vi "CursorReturnForce.vi"(6 "Enable":bool, 8 "ReturnForce":dbl, 9 "Test Name":string(combo)="WDW", 10 "XYGRF_Up":refnum<vi>, 11 "XYGRF_Down":refnum<vi>) -> ()   [LabVIEW 2017]
panel:
  out "DoorLockGraph 2":cluster{"Y":dbl[], "Y":dbl[]}[](graph)
  out "DoorLockGraph":cluster{"Y":dbl[], "Y":dbl[]}[](graph)
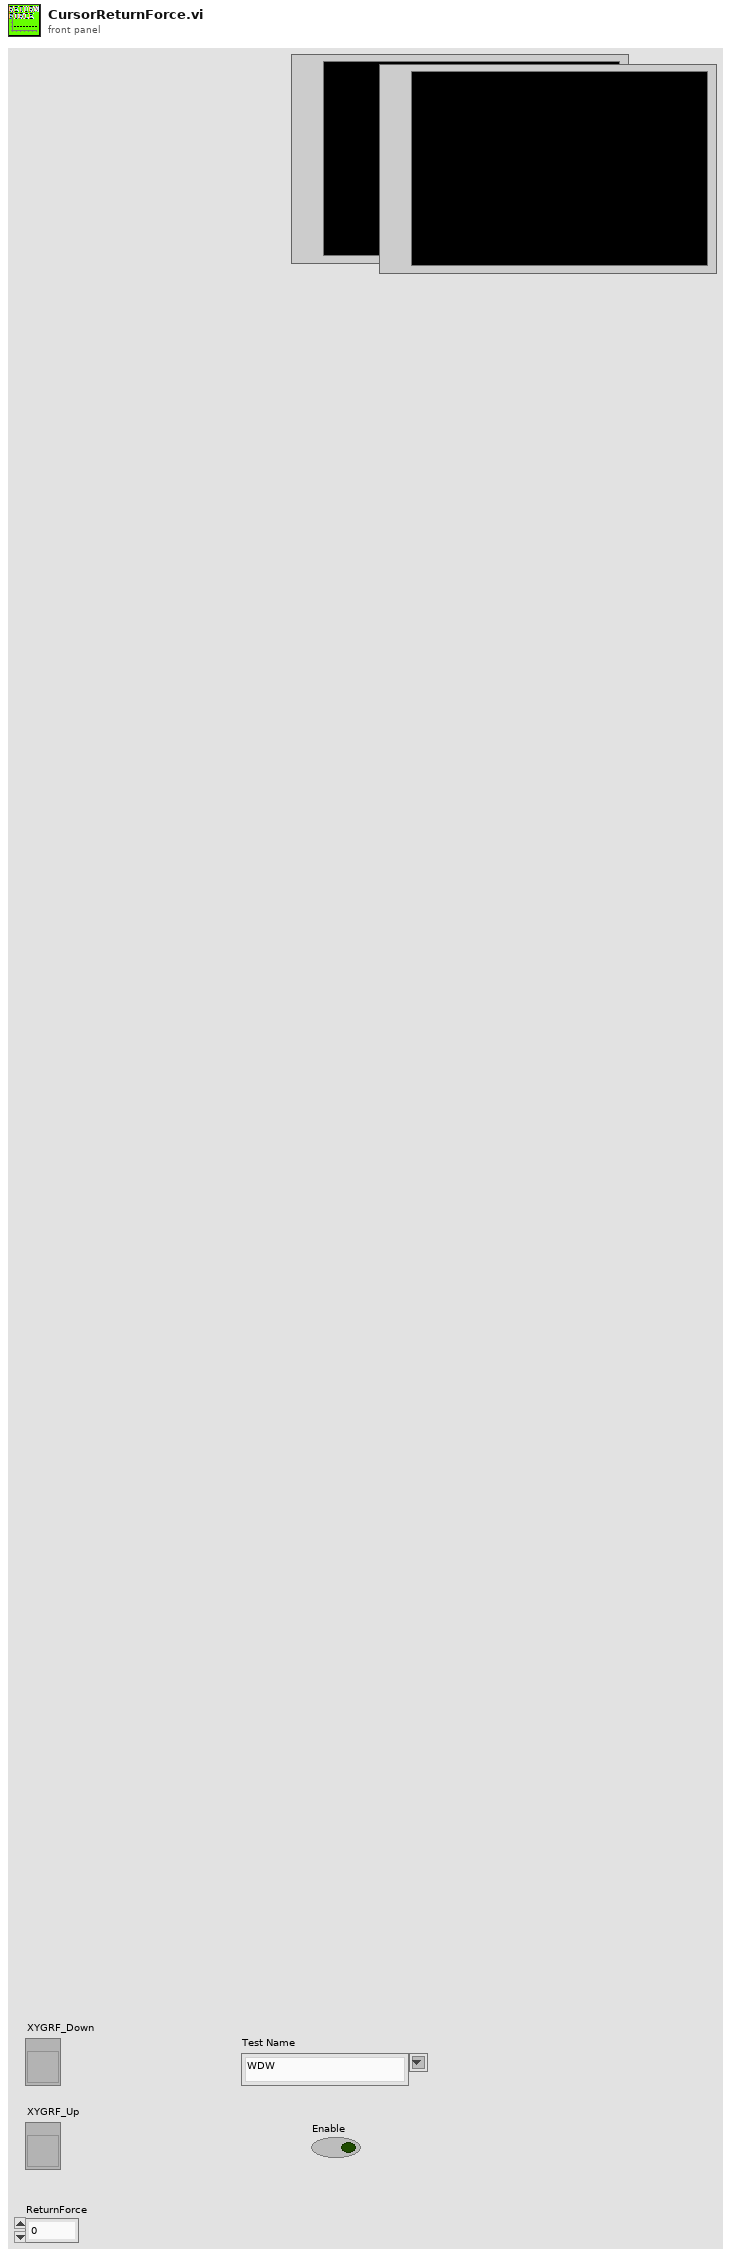
[diagram p1: front panel]
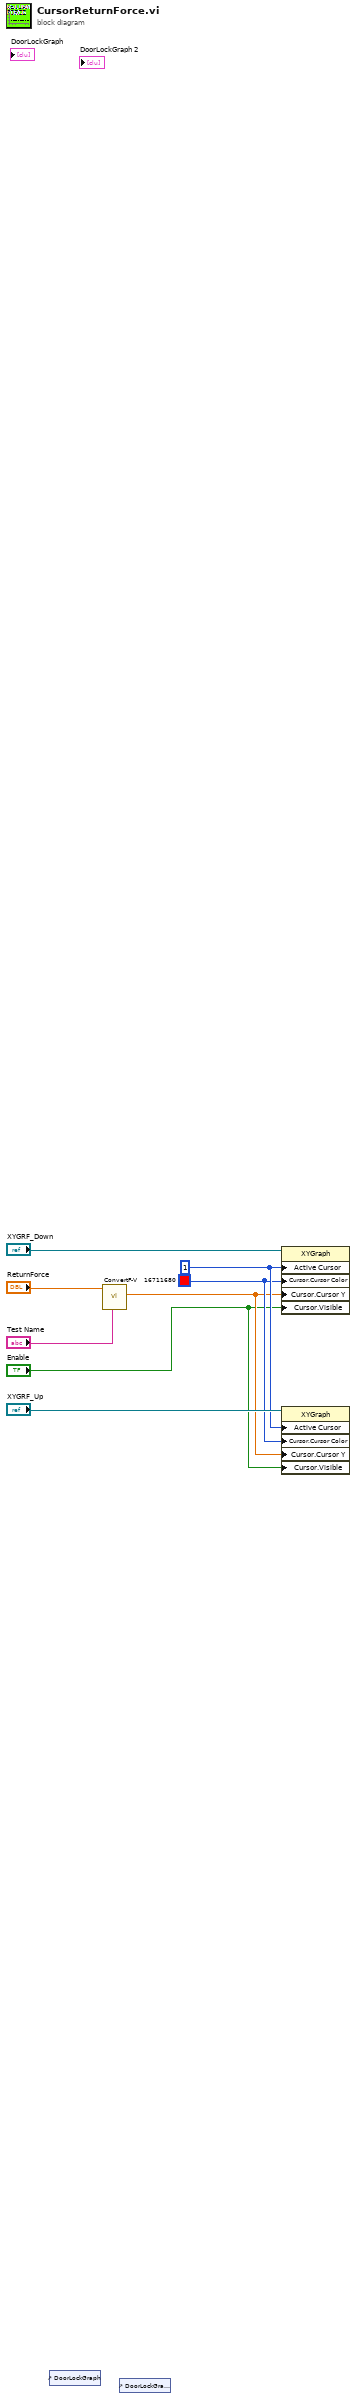
[diagram p0: block diagram]
diagram:
  w3 = u32 16711680
  w4 = u32 1 ("Active Cursor")
  n1 = control-ref of="DoorLockGraph"() -> ()  [unwired: 1 out]
  n2 = call "ConvertF-V.vi"("Test Name"="Test Name", "Force  Spect"="ReturnForce") -> ("F-V Normal"=w2:dbl)  [unwired: 7 in, 2 out]
  n3 = control-ref of="DoorLockGraph 2"() -> ()  [unwired: 1 out]
  n4 = property class="XYGraph"(reference="XYGRF_Down", "Active Cursor"=w4, "Cursor.Cursor Color"=w3, "Cursor.Cursor Y"=w2, "Cursor.Visible"="Enable") -> ()  [unwired: 1 in, 2 out]
  n5 = property class="XYGraph"(reference="XYGRF_Up", "Active Cursor"=w4, "Cursor.Cursor Color"=w3, "Cursor.Cursor Y"=w2, "Cursor.Visible"="Enable") -> ()  [unwired: 1 in, 2 out]
